vi "LocalAppData Build Path.vi"(8 "error in (no error)":errorcluster, 11 "Relative path":path) -> (0 "error out":errorcluster, 3 "Full Path":path)   [LabVIEW 2020, in "RxnRover.lvlib" / "File IO.lvlib" / "LocalAppData Utilities.lvlib"]
doc: "Builds a file path with relative path and Local App Data Base Path\nAn Operating system must be specified\nSupports: Windows 2000 - Windows 11, Linux, Mac OS\n\nCreated 5/20/2025 - Labview 2020\nRxnRover"
uses:
  LocalAppData Utilities.lvlib
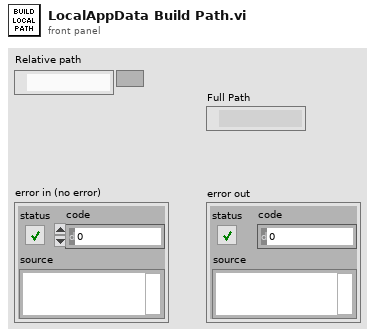
[diagram p1: front panel]
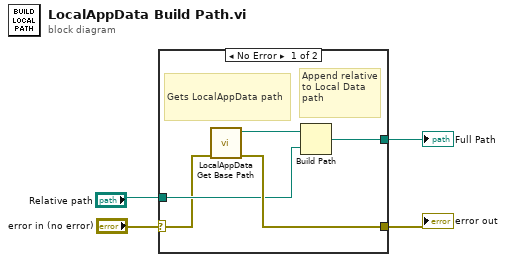
[diagram p0: block diagram]
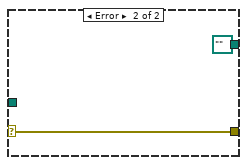
[diagram p2: hidden frame]
diagram:
  n1 = case shown="No Error" "error in (no error)" {
    selector: "error in (no error)" -> [w5 w11]
    tunnel: [w9 w11] -> w4
    tunnel: [w8 path "" ("appended path")] -> w3
    tunnel: "Relative path" -> [w6 _]
    frame No Error {
      # "Gets LocalAppData path"
      # "Append relative to Local Data path"
      n2 = call "LocalAppData Get Base Path.vi"("error in (no error)"=w5) -> ("error out"=w9:errorcluster, "Path"=w7:path)  [unwired: 9 in]
      n3 = Build Path(base path=w7, name or relative path=w6) -> (appended path=w8:path)
    }
    frame Error {
    }
  }
  "error out" <- w4
  "Full Path" <- w3
